vi "omni with motors.vi"   [LabVIEW 2010, in "Omni2013.lvrbt"]
uses:
  Omni2013.lvrbt
  <vilib>/NXT/Dual Mode Library/Motors/Rotation.vi
  <vilib>/NXT/Dual Mode Library/Display/drawNumber_float.vi
types:
  T1 = typedef "LVHSConnector.ctl" = cluster{"Hardware":string, "Flattened String":string}
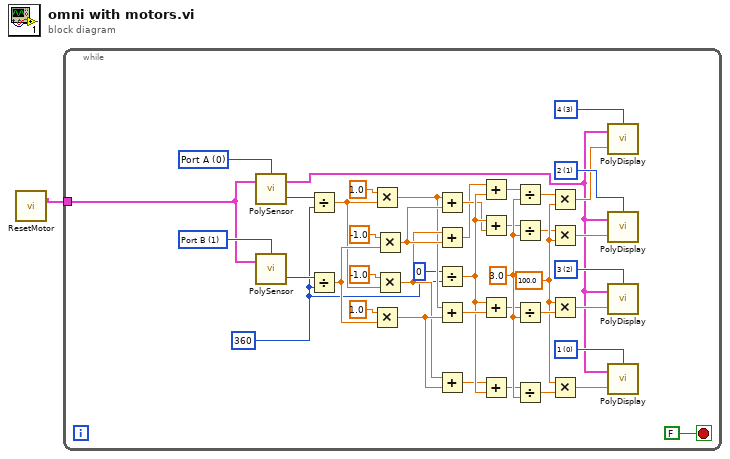
[diagram p0: block diagram]
diagram:
  n1 = call <vilib>:"ResetMotor.vi"() -> ("NXT"=w1:T1)  [unwired: 4 in]
  n2 = while {
    tunnel: w1 -> [w3]
    stop <- FALSE stop-if-true
    w2 = 360
    w8 = u8 1 items=["Port A", "Port B", "Port C"] ("Port (Port A)")
    w10 = u8 0 items=["Port A", "Port B", "Port C"] ("Port (Port A)")
    w43 = i16 0 items=["1", "2", "3", "4", "5", "6", "7", "8"] ("Line")
    w42 = i16 3 items=["1", "2", "3", "4", "5", "6", "7", "8"] ("Line")
    w13 = i16 2 items=["1", "2", "3", "4", "5", "6", "7", "8"] ("Line")
    w41 = i16 1 items=["1", "2", "3", "4", "5", "6", "7", "8"] ("Line")
    w36 = 100.0 ("y")
    w39 = 3.0 ("y")
    n3 = call-poly <vilib>:"PolySensor.vi"("NXT"=w3, "Port (Port A)"=w10) -> ("Angle of Rotation"=w9:i32, "NXT"=w6:T1)  [unwired: 1 in]
    n4 = call-poly <vilib>:"PolySensor.vi"("NXT"=w3, "Port (Port A)"=w8) -> ("Angle of Rotation"=w7:i32)  [unwired: 1 in, 1 out]
    n5 = Divide(x=w9, y=w2) -> (x/y=w18:dbl)
    n6 = Divide(x=w7, y=w2) -> (x/y=w21:dbl)
    n7 = Multiply(x=1.0, y=w18) -> (x*y=w22:dbl)
    n8 = Multiply(x=1.0, y=w21) -> (x*y=w37:dbl)
    n9 = Multiply(x=-1.0, y=w21) -> (x*y=w24:dbl)
    n10 = Multiply(x=-1.0, y=w18) -> (x*y=w23:dbl)
    n11 = Add(x=w22, y=w24) -> (x+y=w26:dbl)
    n12 = Add(x=w23, y=w24) -> (x+y=w25:dbl)
    n13 = Divide(x=i8 0, y=w2) -> (x/y=w31:dbl)
    n14 = Add(x=w22, y=w37) -> (x+y=w38:dbl)
    n15 = Add(x=w23, y=w37) -> (x+y=w27:dbl)
    n16 = Add(x=w25, y=w31) -> (x+y=w30:dbl)
    n17 = Add(x=w31, y=w26) -> (x+y=w29:dbl)
    n18 = Add(x=w31, y=w38) -> (x+y=w32:dbl)
    n19 = Add(x=w27, y=w31) -> (x+y=w28:dbl)
    n20 = Divide(x=w30, y=w39) -> (x/y=w33:dbl)
    n21 = Divide(x=w29, y=w39) -> (x/y=w34:dbl)
    n22 = Divide(x=w32, y=w39) -> (x/y=w40:dbl)
    n23 = Divide(x=w28, y=w39) -> (x/y=w35:dbl)
    n24 = Multiply(x=w33, y=w36) -> (x*y=w12:dbl)
    n25 = Multiply(x=w34, y=w36) -> (x*y=w14:dbl)
    n26 = Multiply(x=w36, y=w40) -> (x*y=w11:dbl)
    n27 = Multiply(x=w36, y=w35) -> (x*y=w15:dbl)
    n28 = call-poly <vilib>:"PolyDisplay.vi"("number"=w12, "NXT"=w6, "Line"=w42) -> ()  [unwired: 1 in, 1 out]
    n29 = call-poly <vilib>:"PolyDisplay.vi"("number"=w14, "NXT"=w6, "Line"=w41) -> ()  [unwired: 1 in, 1 out]
    n30 = call-poly <vilib>:"PolyDisplay.vi"("number"=w11, "NXT"=w6, "Line"=w13) -> ()  [unwired: 1 in, 1 out]
    n31 = call-poly <vilib>:"PolyDisplay.vi"("number"=w15, "NXT"=w6, "Line"=w43) -> ()  [unwired: 1 in, 1 out]
  }
